vi "Ejercicio4_Depuracion.vi"() -> ()   [LabVIEW 2022 SP3]
panel:
  out "Resultado":dbl
  in  "Control":dbl
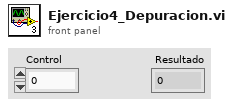
[diagram p1: front panel]
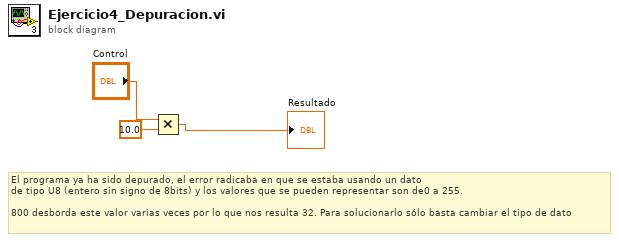
[diagram p0: block diagram]
diagram:
  # "El programa ya ha sido depurado, el error radicaba en que se estaba usando un dato\nde tipo U8 (entero sin signo de 8bits) y los valores que se pueden representar son de0 a 255.\n\n800 desborda este valor varias veces por lo que nos resulta 32. Para solucionarlo sólo basta cambiar el tipo de dato"
  n1 = Multiply(x="Control", y=10.0) -> (x*y=→"Resultado":dbl)
